vi "Count weekdays.vi"(1 "Days":i32[](array[numeric])) -> (0 "Day counts":i32[](array[numeric]))   [LabVIEW 2015]
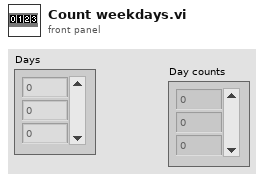
[diagram p1: front panel]
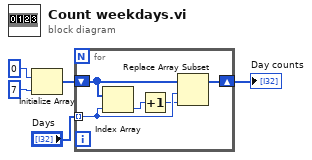
[diagram p0: block diagram]
diagram:
  n1 = Initialize Array(0 ("Numeric"), 7 ("dimension size")) -> (w1:i32[])
  n2 = for {
    tunnel: "Days" -> [w9] mode=indexing
    shift-right: [w6] -> w4
    shift-left: w1 -> [w10]
    n3 = Index Array(array=w10, index=w9) -> (element=w8:i32)
    n4 = Increment(x=w8) -> (x+1=w7:i32)
    n5 = Replace Array Subset(array=w10, new element=w7, index=w9) -> (w6:i32[])
  }
  "Day counts" <- w4
